vi "Get Variant.vi"(8 "error in (no error)":errorcluster, 11 "int32 in":refnum<class "int32.lvclass">) -> (0 "error out":errorcluster, 2 "Variant":variant, 3 "int32 out":refnum<class "int32.lvclass">)   [LabVIEW 2020, in "Protobuf RAW.lvlib" / "int32.lvclass"]
uses:
  int32.lvclass
  int32.lvclass/int32.ctl
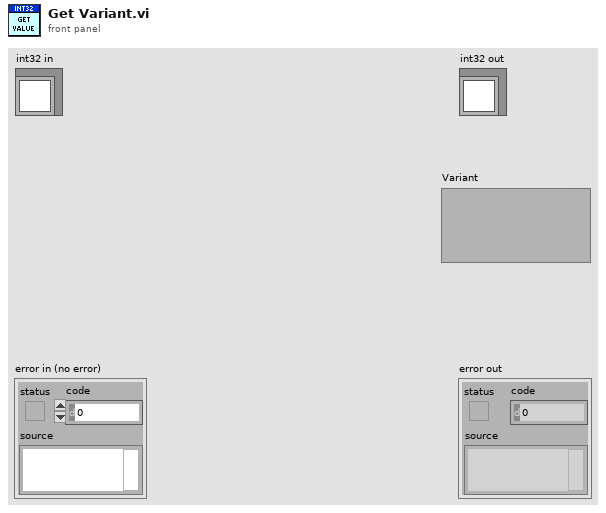
[diagram p1: front panel]
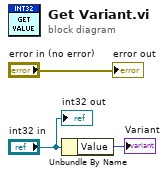
[diagram p0: block diagram]
diagram:
  n1 = Unbundle By Name("int32 in") -> ("Value"=→"Variant":i32)
  "error out" <- "error in (no error)"
  "int32 out" <- "int32 in"
